vi "StopCW.vi"(6 "Resp Timeout (ms)":i32 min=0, 7 "Enum":T1, 8 "Error In":errorcluster, 11 "FPGA Reference":refnum<k20>) -> (0 "Error Out":errorcluster, 1 "Received Text":string, 2 "Stop CW OK":bool)   [LabVIEW 2018]
uses:
  Resources_Test/UART/ControlTestSlot.ctl
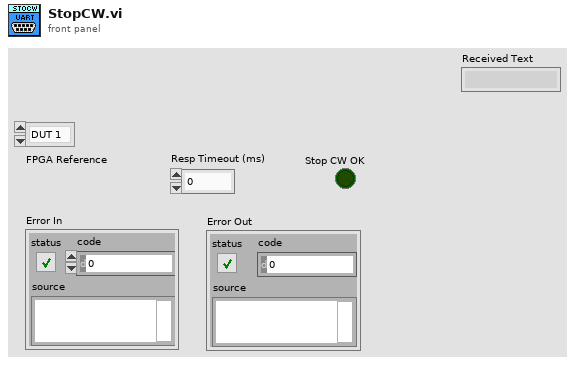
[diagram p1: front panel]
types:
  T1 = typedef "ControlTestSlot.ctl" = enum16{"DUT 1", "DUT 2"}
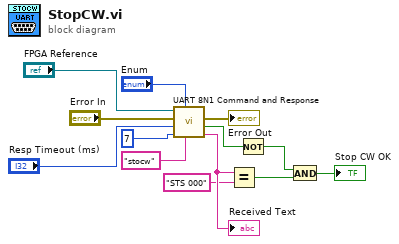
[diagram p0: block diagram]
diagram:
  n1 = call "UART 8N1 Command and Response.vi"("Text to Send"="stocw", "Active Dut"="Enum", "Response Size (char)"=u32 7, "Response Timeout (ms)"="Resp Timeout (ms)", "Error In"="Error In", "FPGA VI Reference In"="FPGA Reference") -> ("Received Text"=w2:string, "Timeout Flag"=w3:bool, "Error Out"=→"Error Out":errorcluster)  [unwired: 1 in, 2 out]
  "Received Text" <- w2
  n2 = Equal?(x=w2, y="STS 000") -> (x = y?=w12:bool)
  n3 = Not(x=w3) -> (.not. x?=w13:bool)
  n4 = And(x=w13, y=w12) -> (x .and. y?=→"Stop CW OK":bool)
